vi "Write Binary Config.vi"(4 "Include Class Name":bool, 6 "byte order (0:big-endian, network order)":T1(ring), 8 "error in (no error)":errorcluster, 11 "Subset_STR in":refnum<class "Subset_STR.lvclass">) -> (0 "error out":errorcluster, 2 "Binary":string, 3 "Subset_STR out":refnum<class "Subset_STR.lvclass">)   [LabVIEW 2021, in "Subset_STR.lvclass"]
uses:
  Subset_STR.lvclass
  Subset_STR.lvclass/Subset_STR.ctl
  Abs_Types/String/Abs_String.lvclass
  Abs_Types/Numeric/Abs_Numeric.lvclass
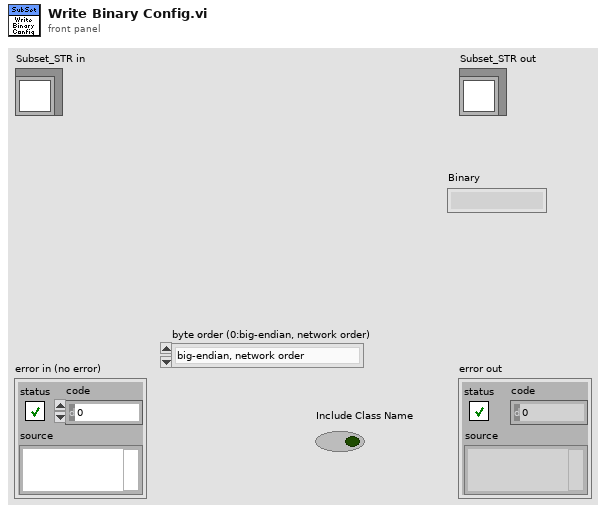
[diagram p1: front panel]
types:
  T1 = enum16{"big-endian, network order", "native, host order", "little-endian"}
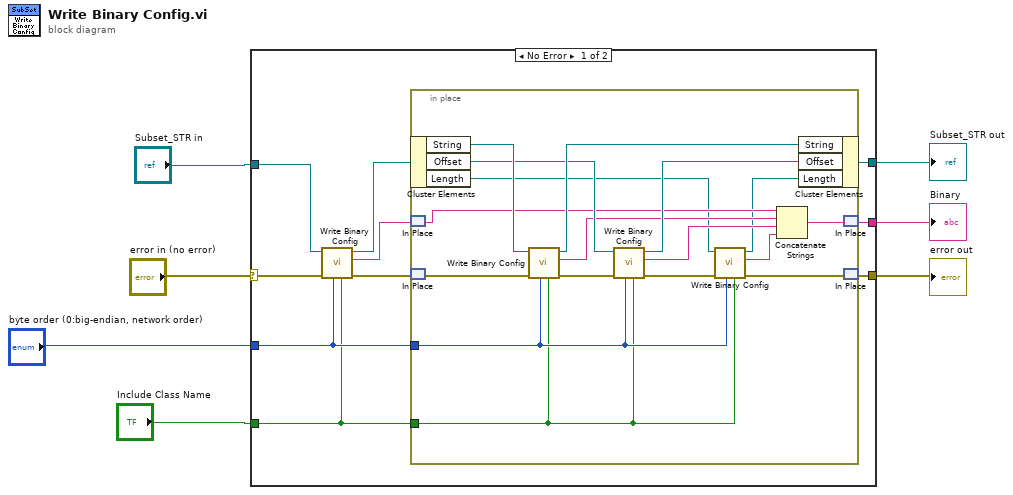
[diagram p0: block diagram]
diagram:
  n1 = case shown="No Error" "error in (no error)" {
    selector: "error in (no error)" -> [w17 w35]
    tunnel: "Subset_STR in" -> [w16 w36]
    tunnel: [w12 _] -> w2
    tunnel: "byte order (0:big-endian, network order)" -> [w11 _]
    tunnel: "Include Class Name" -> [w10 _]
    tunnel: [w9 w35] -> w6
    tunnel: [w8 w36] -> w1
    frame No Error {
      n2 = call-parent "Write Binary Config.vi"("Include Class Name"=w10, "byte order (0:big-endian, network order)"=w11, "error in (no error)"=w17, "Abs_Type in"=w16) -> ("error out"=w14:errorcluster, "Binary"=w13:string, "Abs_Type out"=w15:refnum<class "Subset_STR.lvclass">)  [unwired: 5 in]
      n3 = in-place {
        in-place-border: w11 -> [w19]
        in-place-border: w10 -> [w18]
        n4 = in-place-cluster #1(w15) -> ("String"=w32:refnum<class "Abs_String.lvclass">, "Offset"=w31:refnum<class "Abs_Numeric.lvclass">, "Length"=w22:refnum<class "Abs_Numeric.lvclass">)
        n5 = in-place-match #2(w13) -> (w27:string)
        n6 = in-place-match #3(w14) -> (w34:errorcluster)
        n7 = call-dynamic "Write Binary Config.vi"("Include Class Name"=w18, "byte order (0:big-endian, network order)"=w19, "error in (no error)"=w34, "Abs_Type in"=w32) -> ("error out"=w29:errorcluster, "Binary"=w26:string, "Abs_Type out"=w33:refnum<class "Abs_String.lvclass">)  [unwired: 5 in]
        n8 = call-dynamic "Write Binary Config.vi"("Include Class Name"=w18, "byte order (0:big-endian, network order)"=w19, "error in (no error)"=w29, "Abs_Type in"=w31) -> ("error out"=w24:errorcluster, "Binary"=w28:string, "Abs_Type out"=w30:refnum<class "Abs_Numeric.lvclass">)  [unwired: 5 in]
        n9 = call-dynamic "Write Binary Config.vi"("Include Class Name"=w18, "byte order (0:big-endian, network order)"=w19, "error in (no error)"=w24, "Abs_Type in"=w22) -> ("error out"=w23:errorcluster, "Binary"=w20:string, "Abs_Type out"=w21:refnum<class "Abs_Numeric.lvclass">)  [unwired: 5 in]
        n10 = Concatenate Strings(w27, w26, w28, w20) -> (w25:string)
        n11 = in-place-cluster #1("String"=w33, "Offset"=w30, "Length"=w21) -> (w8:refnum<class "Subset_STR.lvclass">)
        n12 = in-place-match #2(w25) -> (w12:string)
        n13 = in-place-match #3(w23) -> (w9:errorcluster)
      }
    }
    frame Error {
    }
  }
  "error out" <- w6
  "Subset_STR out" <- w1
  "Binary" <- w2
